vi "CSV Second Checker.vi"() -> ()   [LabVIEW 2021]
uses:
  <vilib>/Utility/file.llb/Read Delimited Spreadsheet (string).vi
panel:
  in  "Engineering Mode":bool
  out "Error Data Points":string[](array[string])
  out "ERROR DETECTED":bool
  out "String":string
  out "Loop Iteration":i32
  out "Seconds Between Points":i16
  out "Extracted Seconds":i16
  out "match + rest of string":string
  out "substring before match":string
  out "delimited string":string
  out "first subarray":string[](array[string])
  out "array w/ subset deleted":string[](array[string])
  out "deleted portion":string
  out "subarray":string[](array[string])
  out "size(s)":i32
  out "all rows":string[][](array[string])
  out "error out":errorcluster
  in  "File Path":path
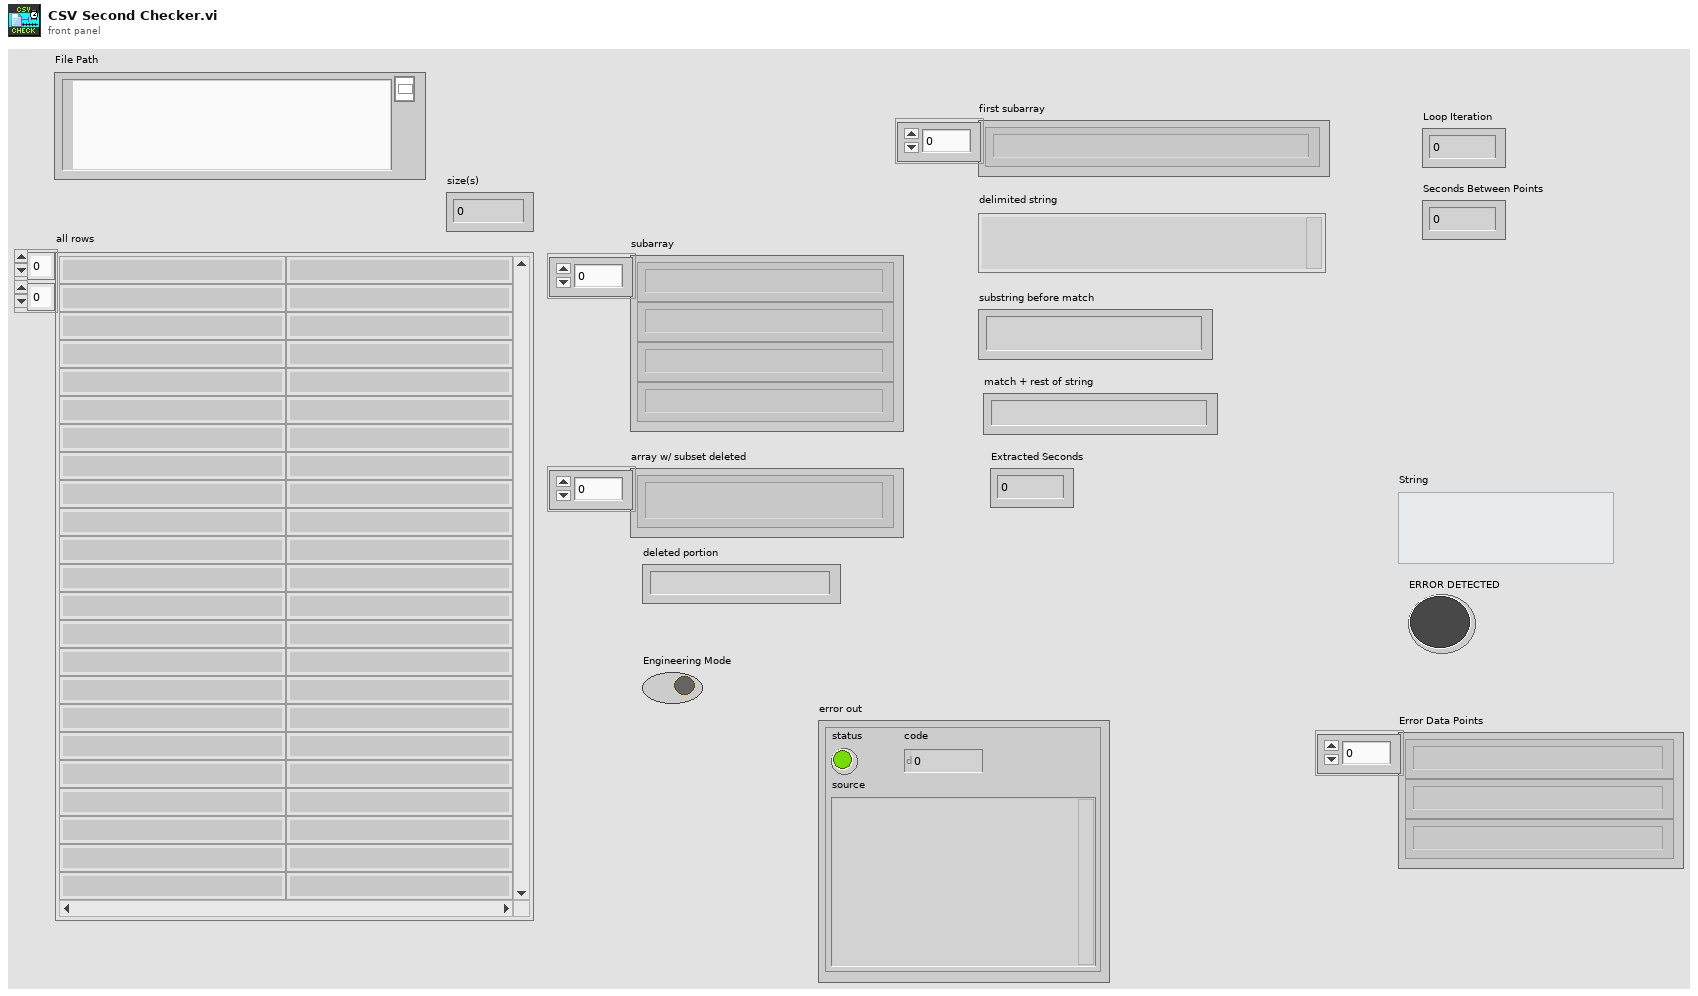
[diagram p1: front panel]
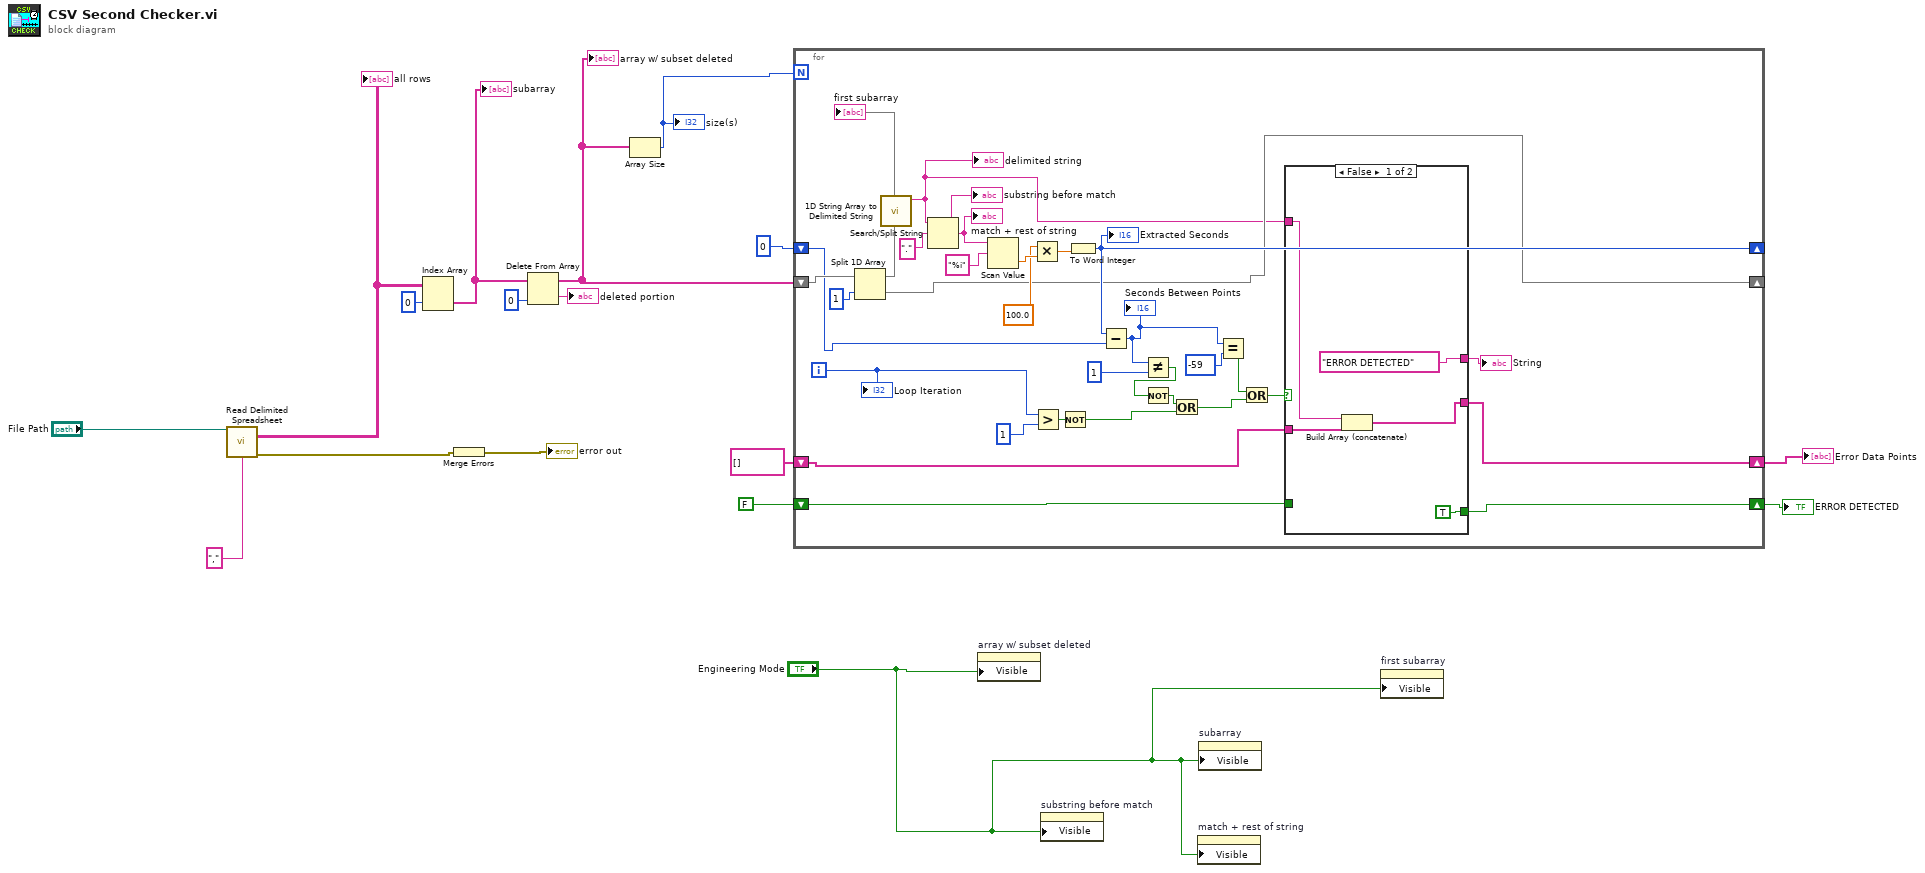
[diagram p0: block diagram]
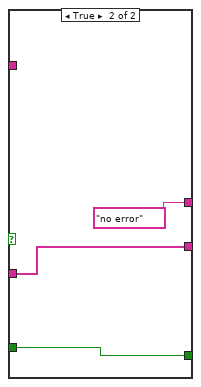
[diagram p2: hidden frame]
diagram:
  n1 = call-poly <vilib>:"Read Delimited Spreadsheet.vi"("file path (dialog if empty)"="File Path", "delimiter (\\t)"="," ("delimiter (\\t)")) -> ("all rows"=w13:string[][], "error out"=w15:errorcluster)  [unwired: 8 in, 4 out]
  "all rows" <- w13
  n2 = Index Array "Index Array"(array=w13, index (col)=0 ("disabled index (col)")) -> (element=w11:string[])  [unwired: 1 in]
  "subarray" <- w11
  n3 = Merge Errors(w15) -> (→"error out":errorcluster)
  n4 = Delete From Array(array=w11, index=0) -> (deleted portion=→"deleted portion":string, array with subset deleted=w8:string[])  [unwired: 1 in]
  "array w/ subset deleted" <- w8
  n5 = Array Size(array=w8) -> (size(s)=w6:i32)
  "size(s)" <- w6
  n6 = for {
    N: w6 -> [_]
    shift-right: [w19] -> _
    shift-left: w8 -> [w48]
    shift-right: [w38] -> _
    shift-left: i16 0 -> [w37]
    shift-right: [w28] -> w3
    shift-left: string[] [] -> [w27]
    shift-right: [w24] -> w4
    shift-left: FALSE -> [w23]
    i -> [w29]
    n7 = Split 1D Array(array=w48, index=1) -> (first subarray=w46:string[], second subarray=w19:string[])
    "first subarray" <- w46
    n8 = call <vilib>:"1D String Array to Delimited String.vi"("string array"=w46) -> ("delimited string"=w18:string)  [unwired: 10 in]
    "delimited string" <- w18
    n9 = Search/Split String(string=w18, search string/char (-)="." ("regular expression")) -> (substring before match=→"substring before match":string, match + rest of string=w43:string)  [unwired: 1 in, 1 out]
    "match + rest of string" <- w43
    n10 = Scan Value(string=w43, format string="%i") -> (value=w41:dbl)  [unwired: 1 in, 1 out]
    n11 = Multiply(x=100.0, y=w41) -> (x*y=w39:dbl)
    n12 = Greater?(x=w29, y=1) -> (0:w36:bool)
    n13 = Not(x=w36) -> (.not. x?=w34:bool)
    n14 = To Word Integer(number=w39) -> (16bit integer=w38:i16)
    "Extracted Seconds" <- w38
    n15 = Subtract(x=w38, y=w37) -> (x-y=w22:i16)
    "Seconds Between Points" <- w22
    n16 = Not Equal?(x=w22, y=i16 1) -> (x != y?=w20:bool)
    n17 = Not(x=w20) -> (.not. x?=w26:bool)
    n18 = Or(x=w26, y=w34) -> (x .or. y?=w31:bool)
    n19 = Equal?(x=w22, y=-59) -> (x = y?=w32:bool)
    n20 = Or(x=w32, y=w31) -> (x .or. y?=w30:bool)
    n21 = case shown="False" w30 {
      tunnel: [w49 w56] -> w28
      tunnel: w27 -> [w50 w56]
      tunnel: ["ERROR DETECTED" ("String") "no error" ("String")] -> w25
      tunnel: [TRUE w54] -> w24
      tunnel: w23 -> [_ w54]
      tunnel: w18 -> [w51 _]
      frame False {
        n22 = Build Array (concatenate)(w51, w50) -> (w49:string[])
      }
      frame True {
      }
    }
    "String" <- w25
    "Loop Iteration" <- w29
  }
  "ERROR DETECTED" <- w4
  "Error Data Points" <- w3
  n23 = property on="array w/ subset deleted" class="Arr (strict)"("Visible"="Engineering Mode") -> ()  [unwired: 2 in, 2 out]
  n24 = property on="substring before match" class="Str"("Visible"="Engineering Mode") -> ()  [unwired: 2 in, 2 out]
  n25 = property on="match + rest of string" class="Str"("Visible"="Engineering Mode") -> ()  [unwired: 2 in, 2 out]
  n26 = property on="subarray" class="Arr (strict)"("Visible"="Engineering Mode") -> ()  [unwired: 2 in, 2 out]
  n27 = property on="first subarray" class="Arr (strict)"("Visible"="Engineering Mode") -> ()  [unwired: 2 in, 2 out]
